vi "_PC_Pub_Command_Ping.vi"(7 "Loop Times":i32=20, 8 "error in (no error)":errorcluster, 11 "PCIP String":string="100.100.0.123") -> (0 "error out":errorcluster={"status"=TRUE, "code"=5004, "source"="Ping TimeOut"})   [LabVIEW 2018]
uses:
  <vilib>/Utility/error.llb/Error Cluster From Error Code.vi
  <vilib>/ErrorRing/Error Ring.xnode
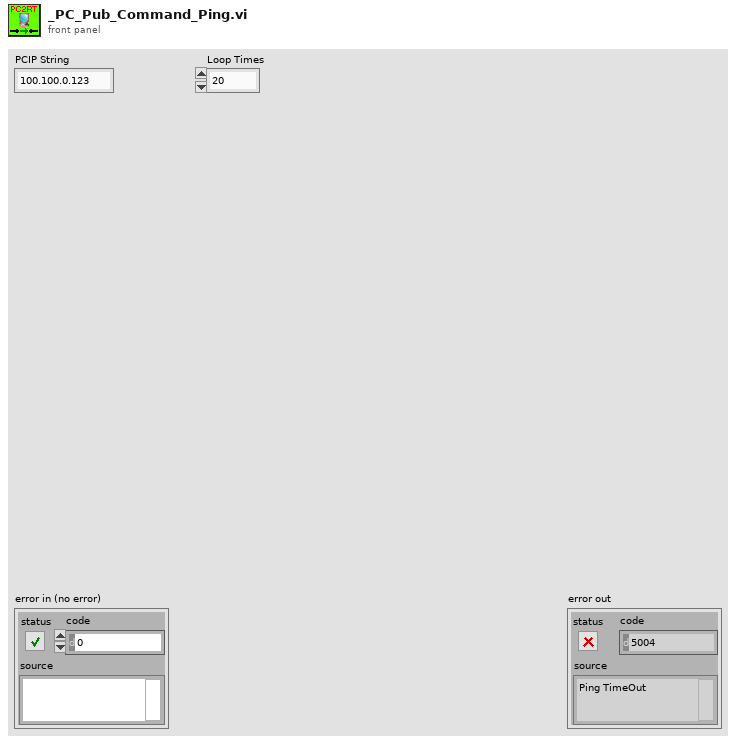
[diagram p1: front panel]
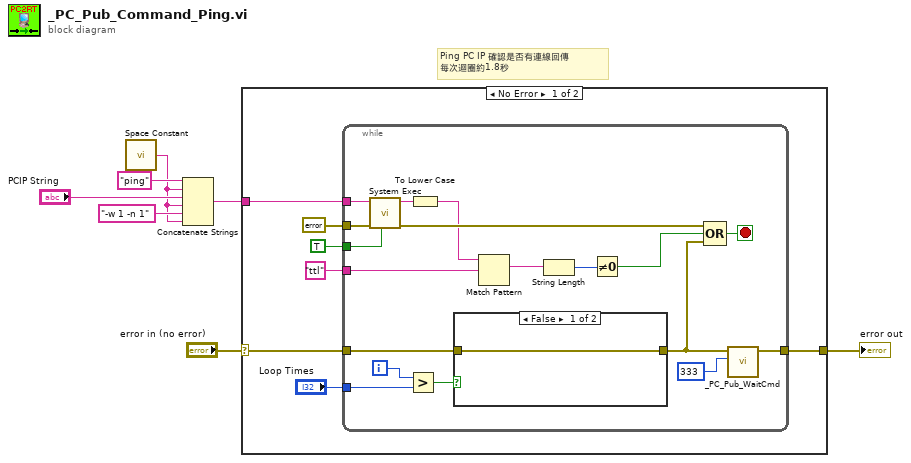
[diagram p0: block diagram]
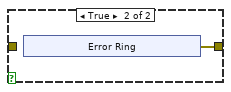
[diagram p2: hidden frame]
diagram:
  # "Ping PC IP 確認是否有連線回傳\n每次迴圈約1.8秒"
  n1 = call <vilib>:"Space Constant.vi"() -> ("String"=w2:string)
  n2 = Concatenate Strings("ping", w2, "PCIP String", w2, "-w 1 -n 1", w2) -> (w1:string)
  n3 = case shown="No Error" "error in (no error)" {
    selector: "error in (no error)" -> [w12 w39]
    tunnel: [w14 w39] -> w6
    tunnel: w1 -> [w9 _]
    frame No Error {
      n4 = while {
        tunnel: w12 -> [w30]
        tunnel: [w16] -> w14
        tunnel: "Loop Times" -> [w29]
        tunnel: errorcluster {"status"=FALSE, "code"=0, "source"=""} ("error in (no error)") -> [w26]
        tunnel: TRUE ("run minimized? (F)") -> [w25]
        tunnel: w9 -> [w24]
        tunnel: "ttl" -> [w19]
        i -> [w32]
        stop <- w27 stop-if-true
        n5 = call <vilib>:"System Exec.vi"("run minimized? (F)"=w25, "error in (no error)"=w26, "command line"=w24) -> ("error out"=w28:errorcluster, "standard output"=w23:string)  [unwired: 5 in, 2 out]
        n6 = Greater?(x=w32, y=w29) -> (0:w31:bool)
        n7 = To Lower Case(string=w23) -> (all lower case string=w18:string)
        n8 = case shown="False" w31 {
          tunnel: w30 -> [w33 _]
          tunnel: [w33 w34] -> w17
          frame False {
          }
          frame True {
            n9 = xnode "Error Ring"() -> ("error out"=w34:errorcluster)
          }
        }
        n10 = Match Pattern(string=w18, regular expression=w19) -> (match substring=w21:string)  [unwired: 1 in, 3 out]
        n11 = String Length(string=w21) -> (length=w22:i32)
        n12 = Not Equal To 0?(x=w22) -> (x != 0?=w20:bool)
        n13 = Compound Arithmetic op=OR(w28, w20, w17) -> (w27:bool)
        n14 = call "_PC_Pub_WaitCmd.vi"("milliseconds to wait"=u32 333, "error in (no error)"=w17) -> ("error out"=w16:errorcluster)  [unwired: 9 in]
      }
    }
    frame Error {
    }
  }
  "error out" <- w6
